vi "NumbOfFingers.vi"(11 "DATA[4]":u8) -> (3 "NumbOfFingers":u8)   [LabVIEW 2020]
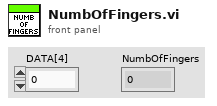
[diagram p1: front panel]
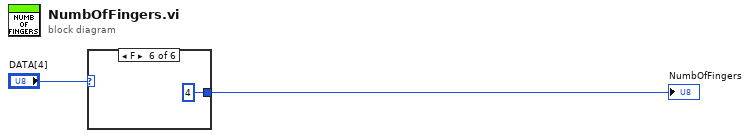
[diagram p0: block diagram]
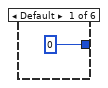
[diagram p2: hidden frame]
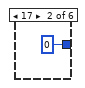
[diagram p3: hidden frame]
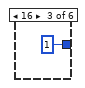
[diagram p4: hidden frame]
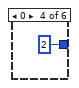
[diagram p5: hidden frame]
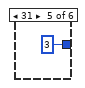
[diagram p6: hidden frame]
diagram:
  n1 = case shown="F" "DATA[4]" {
    tunnel: [u8 0 ("NumbOfFingers") u8 0 ("NumbOfFingers") u8 1 ("NumbOfFingers") u8 2 ("NumbOfFingers") u8 3 ("NumbOfFingers") u8 4 ("NumbOfFingers")] -> w2
    frame Default {
    }
    frame 17 {
    }
    frame 16 {
    }
    frame 0 {
    }
    frame 31 {
    }
    frame 15 {
    }
  }
  "NumbOfFingers" <- w2
